vi "BuildZipName.vi"(11 "Folder":path) -> (3 "Zip File":path)   [LabVIEW 2024]
uses:
  Mic/Mic_Global.vi
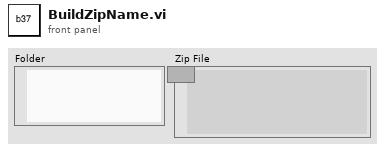
[diagram p1: front panel]
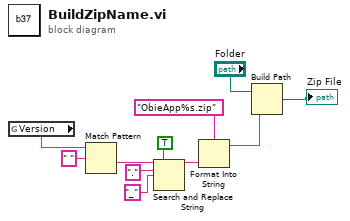
[diagram p0: block diagram]
diagram:
  n1 = global read "Mic_Global.vi" "Version"() -> (w1:string)
  n2 = Match Pattern(string=w1, regular expression=" ") -> (after substring=w3:string)  [unwired: 1 in, 3 out]
  n3 = Search and Replace String(replace all?=TRUE ("replace all? (F)"), input string=w3, search string="." ("regular expression"), replace string="_" ("regular expression")) -> (result string=w7:string)  [unwired: 4 in, 3 out]
  n4 = Format Into String(format string="ObieApp%s.zip" ("regular expression"), w7) -> (resulting string=w9:string)  [unwired: 2 in, 1 out]
  n5 = Build Path(base path="Folder", name or relative path=w9) -> (appended path=→"Zip File":path)
